vi "LINE1_v1.vi"() -> ()   [LabVIEW 2010]
uses:
  <vilib>/express/express arith-compare/Formula/XNode/ExpressFormulaBlockNode.xnode
panel:
  in  "Repetitions":i32
  in  "Current max (mA)":dbl
  in  "wait top (ms)":u32
  in  "wait bottom (ms)":u32
  in  "Motor GPIB":u8=6
  in  "y-dist":u32
  in  "speed":u16
  in  "x-dist":u32
  in  "Current min (mA)":dbl
  in  "Laser GPIB":u8=10 max=100
  out "Dummy":string
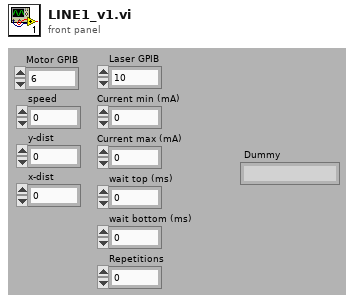
[diagram p1: front panel]
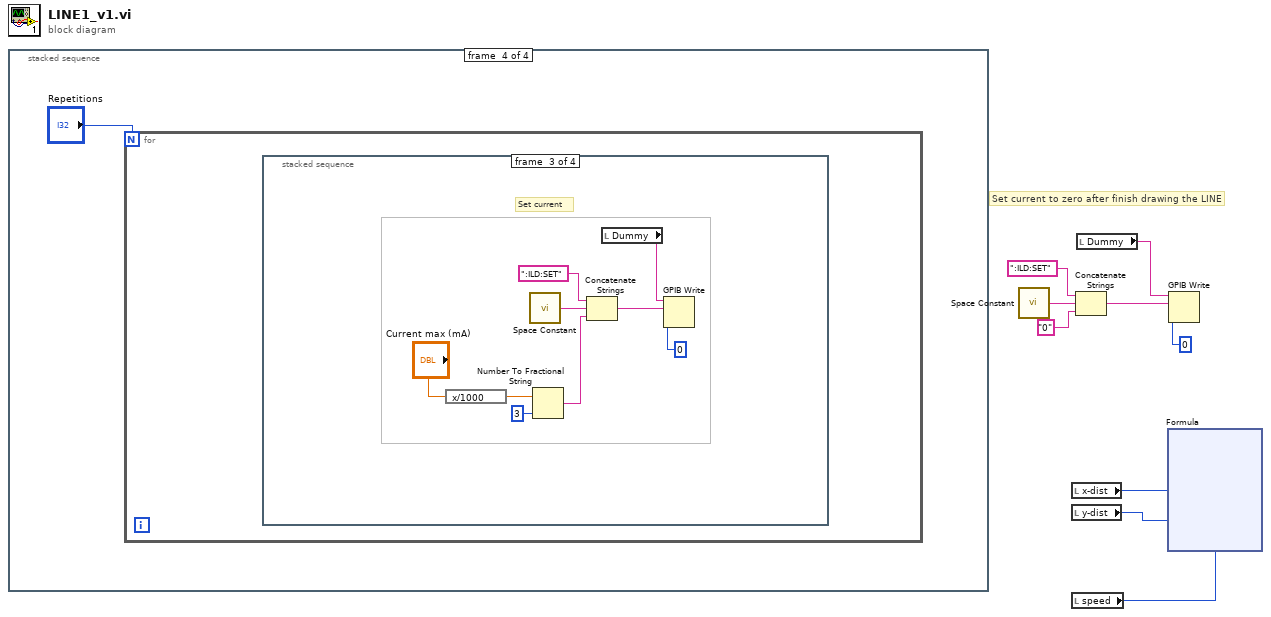
[diagram p0: block diagram]
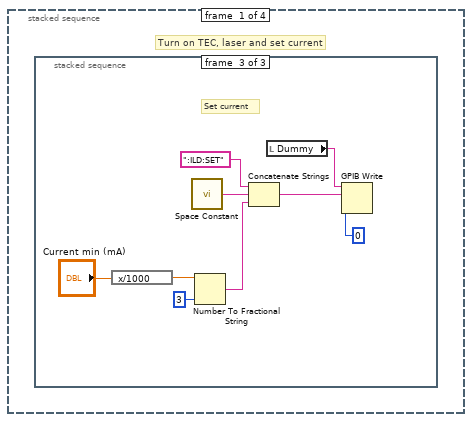
[diagram p2: hidden frame]
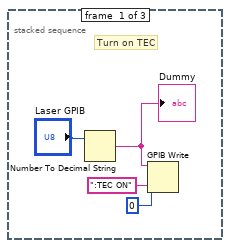
[diagram p3: hidden frame]
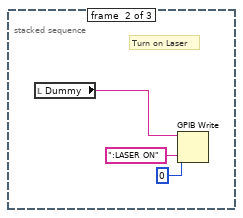
[diagram p4: hidden frame]
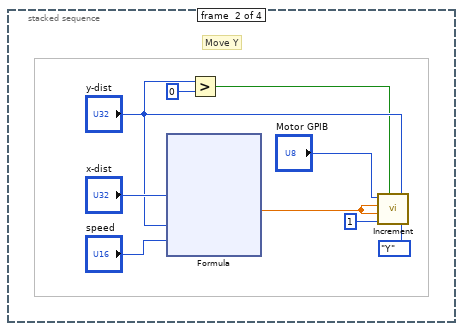
[diagram p5: hidden frame]
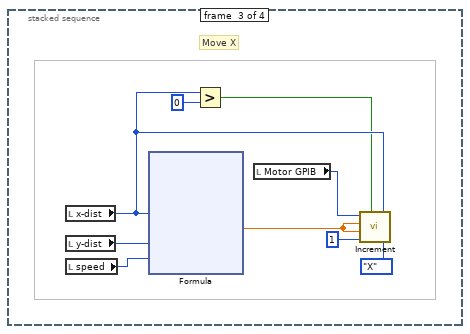
[diagram p6: hidden frame]
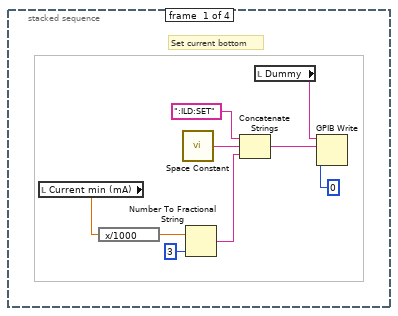
[diagram p7: hidden frame]
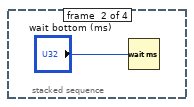
[diagram p8: hidden frame]
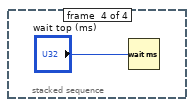
[diagram p9: hidden frame]
diagram:
  # "Set current to zero after finish drawing the LINE"
  n1 = stacked-sequence {
    frame #0 {
      # "Turn on TEC, laser and set current"
      n2 = stacked-sequence {
        frame #0 {
          # "Turn on TEC"
          n3 = Number To Decimal String(number="Laser GPIB") -> (decimal integer string=w10:string)  [unwired: 1 in]
          "Dummy" <- w10
          n4 = GPIB Write(0:w10, 1:":TEC ON" ("data"), 2:i16 0 ("mode (0)")) -> ()  [unwired: 2 in, 2 out]
        }
        frame #1 {
          # "Turn on Laser"
          n5 = local read "Dummy"() -> (w14:string)
          n6 = GPIB Write(0:w14, 1:":LASER ON" ("data"), 2:i16 0 ("mode (0)")) -> ()  [unwired: 2 in, 2 out]
        }
        frame #2 {
          # "Set current"
          n7 = expression code="x/1000"("Current min (mA)") -> (w21:dbl)
          n8 = call <vilib>:"Space Constant.vi"() -> ("String"=w23:string)
          n9 = Number To Fractional String(number=w21, precision (6)=i16 3) -> (F-format string=w18:string)  [unwired: 2 in]
          n10 = Concatenate Strings(":ILD:SET", w23, w18) -> (w22:string)
          n11 = local read "Dummy"() -> (w17:string)
          n12 = GPIB Write(0:w17, 1:w22, 2:i16 0 ("mode (0)")) -> ()  [unwired: 2 in, 2 out]
        }
      }
    }
    frame #1 {
      # "Move Y"
      n13 = xnode "Formula"("X1"="x-dist", "X2"="y-dist", "X3"="speed") -> ("Result"=w29:dbl)  [unwired: 1 in, 1 out]
      n14 = Greater?(x="y-dist", y=u32 0) -> (0:w26:bool)
      n15 = call "Increment.vi"("GPIB_Addr"="Motor GPIB", "F Speed"=w29, "L Speed"=w29, "Rate"=u16 1, "CCW 3"=w26, "Distance"="y-dist", "Axis"=enum16{"X", "Y", "Z", "U", "V", "W"}."Y") -> ()
    }
    frame #2 {
      # "Move X"
      n16 = local read "x-dist"() -> (w49:u32)
      n17 = local read "y-dist"() -> (w52:u32)
      n18 = local read "speed"() -> (w51:u16)
      n19 = xnode "Formula"("X1"=w49, "X2"=w52, "X3"=w51) -> ("Result"=w53:dbl)  [unwired: 1 in, 1 out]
      n20 = Greater?(x=w49, y=u32 0) -> (0:w47:bool)
      n21 = local read "Motor GPIB"() -> (w50:u8)
      n22 = call "Increment.vi"("GPIB_Addr"=w50, "F Speed"=w53, "L Speed"=w53, "Rate"=u16 1, "CCW 3"=w47, "Distance"=w49, "Axis"=enum16{"X", "Y", "Z", "U", "V", "W"}."X") -> ()
    }
    frame #3 {
      n23 = for {
        N: "Repetitions" -> [_]
        n24 = stacked-sequence {
          frame #0 {
            # "Set current bottom"
            n25 = local read "Current min (mA)"() -> (w77:dbl)
            n26 = expression code="x/1000"(w77) -> (w73:dbl)
            n27 = call <vilib>:"Space Constant.vi"() -> ("String"=w71:string)
            n28 = Number To Fractional String(number=w73, precision (6)=i16 3) -> (F-format string=w75:string)  [unwired: 2 in]
            n29 = Concatenate Strings(":ILD:SET", w71, w75) -> (w72:string)
            n30 = local read "Dummy"() -> (w76:string)
            n31 = GPIB Write(0:w76, 1:w72, 2:i16 0 ("mode (0)")) -> ()  [unwired: 2 in, 2 out]
          }
          frame #1 {
            n32 = Wait (ms)(milliseconds to wait="wait bottom (ms)") -> ()  [unwired: 1 out]
          }
          frame #2 {
            # "Set current"
            n33 = expression code="x/1000"("Current max (mA)") -> (w82:dbl)
            n34 = call <vilib>:"Space Constant.vi"() -> ("String"=w84:string)
            n35 = Number To Fractional String(number=w82, precision (6)=i16 3) -> (F-format string=w80:string)  [unwired: 2 in]
            n36 = Concatenate Strings(":ILD:SET", w84, w80) -> (w83:string)
            n37 = local read "Dummy"() -> (w79:string)
            n38 = GPIB Write(0:w79, 1:w83, 2:i16 0 ("mode (0)")) -> ()  [unwired: 2 in, 2 out]
          }
          frame #3 {
            n39 = Wait (ms)(milliseconds to wait="wait top (ms)") -> ()  [unwired: 1 out]
          }
        }
      }
    }
  }
  n40 = call <vilib>:"Space Constant.vi"() -> ("String"=w6:string)
  n41 = local read "x-dist"() -> (w1:u32)
  n42 = local read "y-dist"() -> (w2:u32)
  n43 = local read "speed"() -> (w3:u16)
  n44 = Concatenate Strings(":ILD:SET", w6, "0" ("string")) -> (w7:string)
  n45 = local read "Dummy"() -> (w9:string)
  n46 = xnode "Formula"("X1"=w1, "X2"=w2, "X3"=w3) -> ()  [unwired: 1 in, 2 out]
  n47 = GPIB Write(0:w9, 1:w7, 2:i16 0 ("mode (0)")) -> ()  [unwired: 2 in, 2 out]
